vi "Prime BSI Check ROI.vi"(7 "PVCam ROI":T1, 13 "Cam Settings Ref":refnum<k24>) -> (4 "Full Chip?":bool, 15 "ROI In Bounds?":bool)   [LabVIEW 2020]
uses:
  Prime BSI Type Defs/Prime BSI ROI.ctl
  Y:/Software/Photometrics/Photometrics LabView Package 2021/Dependencies/PVCamNET.dll
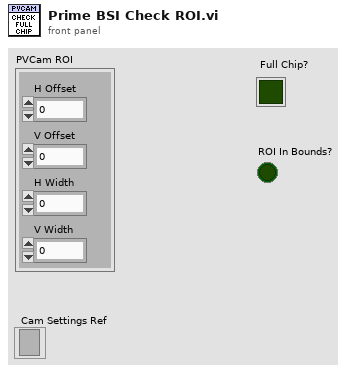
[diagram p1: front panel]
types:
  T1 = typedef "Prime BSI ROI.ctl" = cluster{"H Offset":i32, "V Offset":i32, "H Width":i32, "V Width":i32}
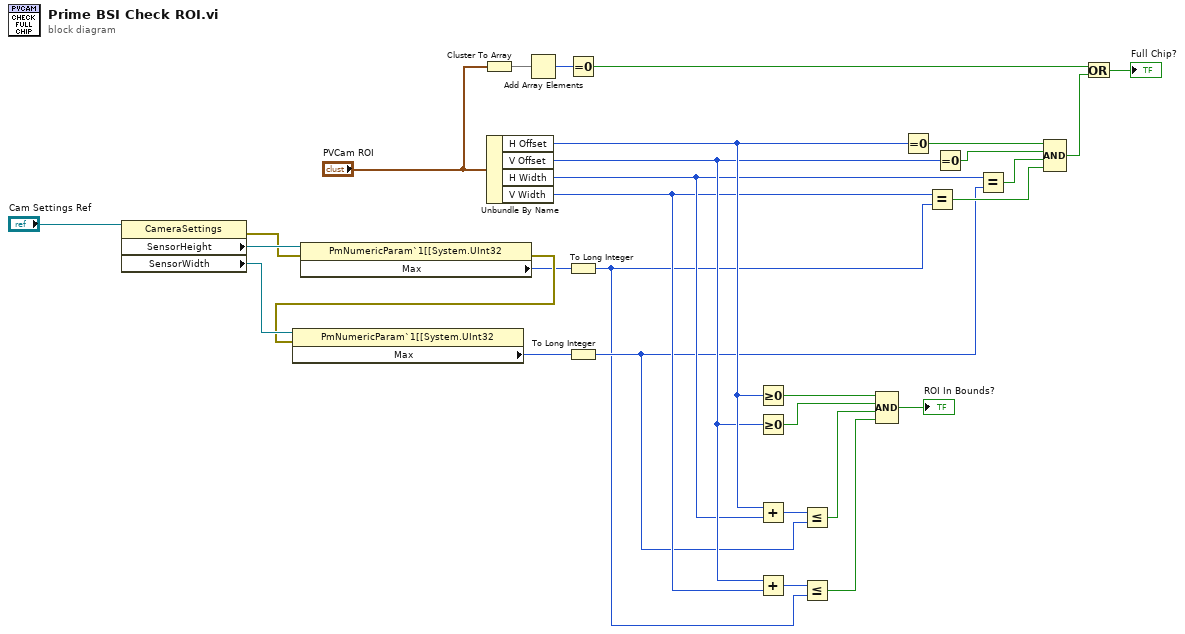
[diagram p0: block diagram]
diagram:
  n1 = property class="CameraSettings"(reference="Cam Settings Ref") -> (error out=w25:errorcluster, "SensorHeight"=w27:refnum<k24>, "SensorWidth"=w26:refnum<k24>)  [unwired: 1 in, 1 out]
  n2 = property class="PmNumericParam`1[[System.UInt32"(reference=w27, error in=w25) -> (error out=w24:errorcluster, "Max"=w22:u32)  [unwired: 1 out]
  n3 = property class="PmNumericParam`1[[System.UInt32"(reference=w26, error in=w24) -> ("Max"=w21:u32)  [unwired: 2 out]
  n4 = Cluster To Array(cluster="PVCam ROI") -> (array=w29:i32[])
  n5 = Unbundle By Name("PVCam ROI") -> ("H Offset"=w13:i32, "V Offset"=w12:i32, "H Width"=w11:i32, "V Width"=w10:i32)
  n6 = Add Array Elements(numeric array=w29) -> (sum=w28:i32)
  n7 = Equal To 0?(x=w28) -> (x = 0?=w16:bool)
  n8 = To Long Integer(number=w22) -> (32bit integer=w6:i32)
  n9 = To Long Integer(number=w21) -> (32bit integer=w8:i32)
  n10 = Greater Or Equal To 0?(x=w13) -> (x >= 0?=w5:bool)
  n11 = Greater Or Equal To 0?(x=w12) -> (x >= 0?=w4:bool)
  n12 = Add(x=w13, y=w11) -> (x+y=w9:i32)
  n13 = Add(x=w12, y=w10) -> (x+y=w7:i32)
  n14 = Less Or Equal?(x=w9, y=w8) -> (x <= y?=w3:bool)
  n15 = Less Or Equal?(x=w7, y=w6) -> (x <= y?=w2:bool)
  n16 = Compound Arithmetic op=AND(w5, w4, w3, w2) -> (→"ROI In Bounds?":bool)
  n17 = Equal To 0?(x=w13) -> (x = 0?=w20:bool)
  n18 = Equal?(x=w10, y=w6) -> (x = y?=w17:bool)
  n19 = Equal To 0?(x=w12) -> (x = 0?=w19:bool)
  n20 = Equal?(x=w11, y=w8) -> (x = y?=w18:bool)
  n21 = Compound Arithmetic op=AND(w20, w19, w18, w17) -> (w15:bool)
  n22 = Or(x=w16, y=w15) -> (x .or. y?=→"Full Chip?":bool)
